vi "Is Late.vi"(8 "error in (no error)":errorcluster, 11 "Transfer Group in":refnum<class "Transfer Group.lvclass">) -> (0 "error out":errorcluster, 3 "Transfer Group out":refnum<class "Transfer Group.lvclass">)   [LabVIEW 2017, in "DSF Core.lvlib" / "Transfer Group.lvclass"]
uses:
  Transfer Group.lvclass
  Transfer Group.lvclass/Transfer Group.ctl
  Return Timeout Error.vi
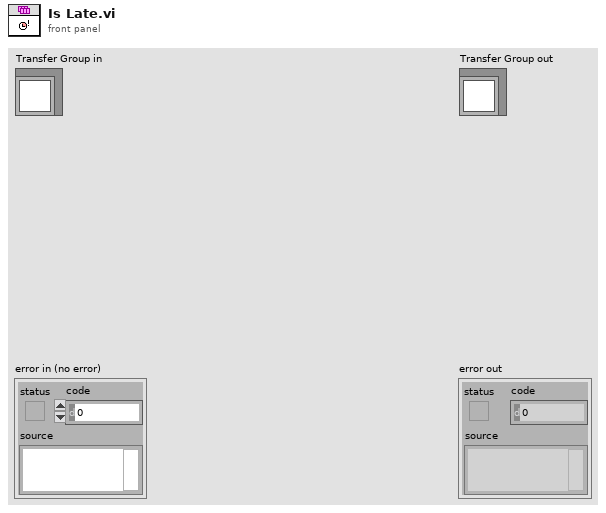
[diagram p1: front panel]
types:
  T1 = typedef "DSF Core.lvlib/DSF Timeout Behavior.ctl" = enum8{"Increment Late Count", "Throw Error"}
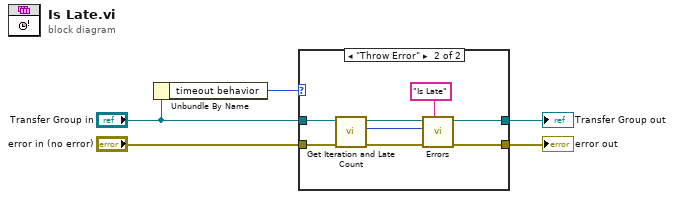
[diagram p0: block diagram]
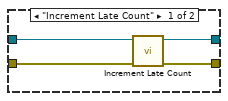
[diagram p2: hidden frame]
diagram:
  n1 = Unbundle By Name("Transfer Group in") -> ("timeout behavior"=w2:T1)
  n2 = case shown="\"Throw Error\"" w2 {
    tunnel: [w8 w17] -> w4
    tunnel: [w9 w16] -> w5
    tunnel: "error in (no error)" -> [w7 w15]
    tunnel: "Transfer Group in" -> [w6 w14]
    frame "Increment Late Count" {
      n3 = call "Increment Late Count.vi"("error in (no error)"=w7, "Transfer Group in"=w6) -> ("error out"=w9:errorcluster, "Transfer Group out"=w8:refnum<class "Transfer Group.lvclass">)  [unwired: 8 in]
    }
    frame "Throw Error" {
      n4 = call "Get Iteration and Late Count.vi"("error in (no error)"=w15, "Transfer Group in"=w14) -> ("error out"=w13:errorcluster, "iteration"=w12:u64, "Transfer Group out"=w11:refnum<class "Transfer Group.lvclass">)  [unwired: 6 in, 1 out]
      n5 = call-poly "Errors.vi"("error source vi name"="Is Late", "error in (no error)"=w13, "iteration"=w12, "Transfer Group in"=w11) -> ("error out"=w16:errorcluster, "Transfer Group out"=w17:refnum<class "Transfer Group.lvclass">)  [unwired: 6 in]
    }
  }
  "error out" <- w5
  "Transfer Group out" <- w4
